vi "Arduino Start Comms.vi"(1 "Resource index":i32, 2 "Arduino VISA config & resource":T1={"VISA resource name"="COM12", "baud rate (bps)"=276000, "timeout (ms)"=12000, "data bits"=8, "parity"=enum."None", "stop bits (10: 1 bit)"=10, "flow control"=0, "termination char (hex)"=10, "Enable Termination Char"=FALSE, "byte count"=12, "Resource locked?"=FALSE} {"termination char (hex)" format="%02x"; "stop bits (10: 1 bit)" items=["1.0"=10, "1.5"=15, "2.0"=20]; "flow control" items=["None", "XON/XOFF", "RTS/CTS", "XON/XOFF & RTS/CTS", "DTR/DSR", "XON/XOFF & DTR/DSR"]}) -> (0 "Error":errorcluster)   [LabVIEW 2013]
uses:
  ctls_and_globals/Arduino Config & resource typedef.ctl
  ctls_and_globals/Arduino Global.vi
  <vilib>/Instr/_visa.llb/VISA Configure Serial Port (Instr).vi
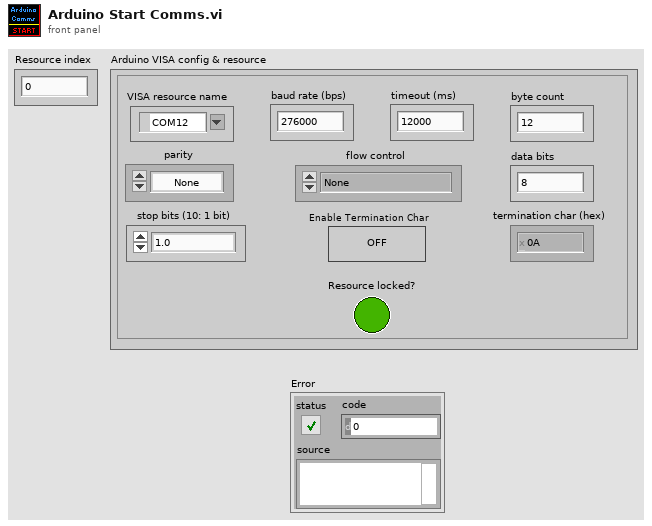
[diagram p1: front panel]
types:
  T1 = typedef "Arduino Config & resource typedef.ctl" = cluster{"VISA resource name":refnum<visa-resource-name>, "baud rate (bps)":u32, "timeout (ms)":u32, "data bits":u16, "parity":enum16{"None", "Odd", "Even", "Mark", "Space"}, "stop bits (10: 1 bit)":u16, "flow control":u16, "termination char (hex)":u8, "Enable Termination Char":bool, "byte count":u32, "Resource locked?":bool}
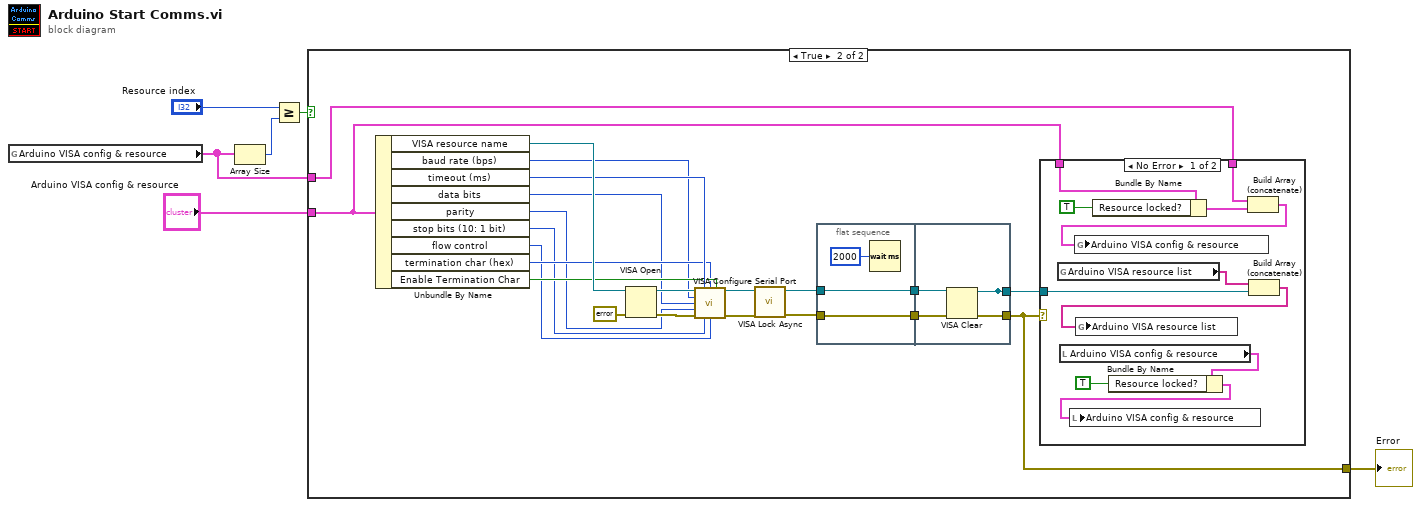
[diagram p0: block diagram]
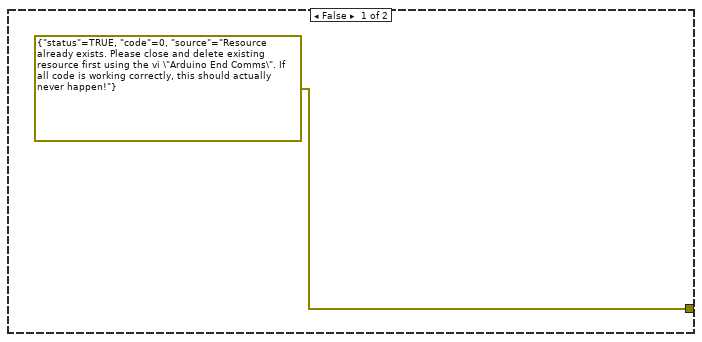
[diagram p2: hidden frame]
diagram:
  n1 = global read "Arduino Global.vi" "Arduino VISA config & resource"() -> (w4:T1[])
  n2 = Array Size(array=w4) -> (size(s)=w6:i32)
  n3 = Greater Or Equal?(x="Resource index", y=w6) -> (x >= y?=w5:bool)
  n4 = case shown="True" w5 {
    tunnel: w4 -> [_ w9]
    tunnel: "Arduino VISA config & resource" -> [_ w11]
    tunnel: [errorcluster {"status"=TRUE, "code"=0, "source"="Resource already exists. Please close and delete existing resource first using the vi \"Arduino End Comms\". If all code is working correctly, this should actually never happen!"} ("error out") w10] -> w2
    frame False {
    }
    frame True {
      n5 = Unbundle By Name(w11) -> ("VISA resource name"=w20:refnum<visa-resource-name>, "baud rate (bps)"=w16:u32, "timeout (ms)"=w19:u32, "data bits"=w15:u16, "parity"=w14:enum16{"None", "Odd", "Even", "Mark", "Space"}, "stop bits (10: 1 bit)"=w13:u16, "flow control"=w12:u16, "termination char (hex)"=w17:u8, "Enable Termination Char"=w18:bool)
      n6 = VISA Open(error in (no error)=errorcluster {"status"=FALSE, "code"=0, "source"=""}, VISA resource name=w20) -> (VISA resource name=w22:refnum<visa-resource-name>, error out=w23:errorcluster)  [unwired: 3 in]
      n7 = call-poly "VISA Configure Serial Port"("VISA resource name"=w22, "timeout (10sec)"=w19, "termination char\n(0xA = '\\n' = LF)"=w17, "Enable Termination\nChar (T)"=w18, "baud rate (9600)"=w16, "data bits (8)"=w15, "parity (0:none)"=w14, "error in (no error)"=w23, "stop bits (10: 1 bit)"=w13, "flow control (0:none)"=w12) -> ("VISA resource name out"=w24:refnum<visa-resource-name>, "error out"=w25:errorcluster)  [unwired: 4 in]
      n8 = call <vilib>:"VISA Lock Async.vi"("error in (no error)"=w25, "VISA resource name"=w24) -> ("error out"=w26:errorcluster, "VISA resource name out"=w27:refnum<visa-resource-name>)  [unwired: 7 in, 1 out]
      n9 = flat-sequence {
        tunnel: w26 -> [w42]
        tunnel: w27 -> [w43]
        tunnel: [w43] -> w28
        tunnel: [w42] -> w29
        tunnel: w29 -> [w46]
        tunnel: w28 -> [w47]
        tunnel: [w44] -> _
        tunnel: [w45] -> w10
        tunnel: [w44] -> w8
        frame #0 {
          n10 = Wait (ms)(milliseconds to wait=u32 2000) -> ()  [unwired: 1 out]
        }
        frame #1 {
          n11 = VISA Clear(VISA resource name=w47, error in (no error)=w46) -> (VISA resource name out=w44:refnum<visa-resource-name>, error out=w45:errorcluster)
        }
      }
      n12 = case shown="No Error" w10 {
        tunnel: w11 -> [w40 _]
        tunnel: w9 -> [w37 _]
        tunnel: w8 -> [w31 _]
        frame No Error {
          n13 = global read "Arduino Global.vi" "Arduino VISA resource list"() -> (w32:string[])
          n14 = local read "Arduino VISA config & resource"() -> (w34:T1)
          n15 = Bundle By Name(cluster=w40, "Resource locked?"=TRUE) -> (w38:T1)
          n16 = Bundle By Name(cluster=w34, "Resource locked?"=TRUE) -> (w33:T1)
          n17 = local write "Arduino VISA config & resource"(w33) -> ()
          n18 = Build Array (concatenate)(w37, w38) -> (w36:T1[])
          n19 = global write "Arduino Global.vi" "Arduino VISA config & resource"(w36) -> ()
          n20 = Build Array (concatenate)(w32, w31) -> (w30:string[])
          n21 = global write "Arduino Global.vi" "Arduino VISA resource list"(w30) -> ()
        }
        frame Error {
        }
      }
    }
  }
  "Error" <- w2
